vi "Read Coupling.vi"(8 "error in (no error)":errorcluster, 11 "Voltage in":refnum<class "Voltage.lvclass">) -> (0 "error out":errorcluster, 2 "Coupling":u16, 3 "Voltage out":refnum<class "Voltage.lvclass">)   [LabVIEW 2018, in "Measurement Channels.lvlib" / "Voltage.lvclass"]
uses:
  Voltage.lvclass
  Voltage.lvclass/Voltage.ctl
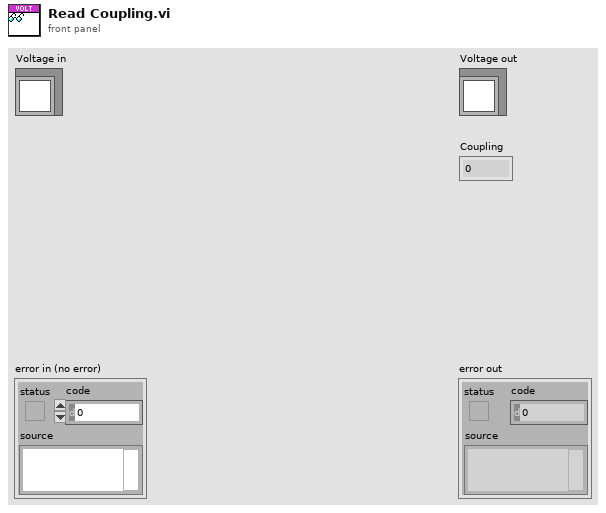
[diagram p1: front panel]
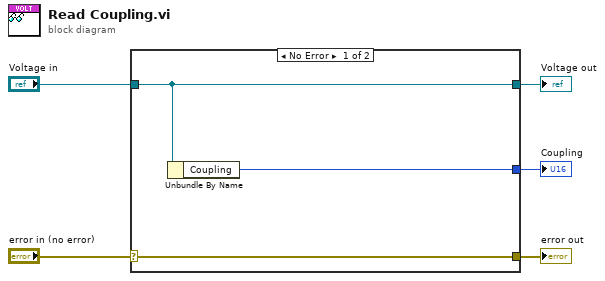
[diagram p0: block diagram]
diagram:
  n1 = case shown="No Error" "error in (no error)" {
    selector: "error in (no error)" -> [w8 w9]
    tunnel: [w8 w9] -> w4
    tunnel: [w7 w10] -> w2
    tunnel: "Voltage in" -> [w7 w10]
    tunnel: [w6 _] -> w1
    frame No Error {
      n2 = Unbundle By Name(w7) -> ("Coupling"=w6:u16)
    }
    frame Error {
    }
  }
  "error out" <- w4
  "Voltage out" <- w2
  "Coupling" <- w1
